vi "Insert Created.vi"(8 "Self":refnum<class "Msg Type Strategy.lvclass">, 9 "Self Alias":string, 10 "Addresses DVR in":refnum<data-value>) -> (0 "error out":errorcluster, 2 "Addresses DVR out":refnum<data-value>)   [LabVIEW 2021, in "jettl.lvlib" / "Addresses.lvlib"]
uses:
  Addresses.lvlib
  Addresses/Addresses.lvclass
  Msg Type Strategy/Msg Type Strategy/Msg Type Strategy.lvclass
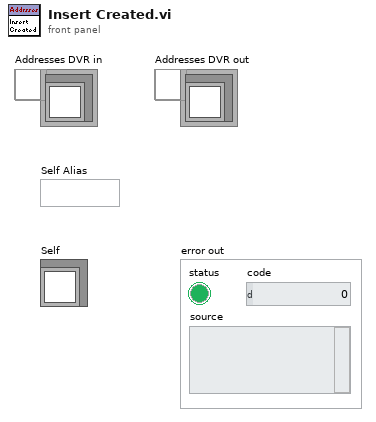
[diagram p1: front panel]
types:
  T1 = typedef "jettl.lvlib/Addresses.lvlib/Created.ctl" = map{string, refnum<class "Msg Type Strategy.lvclass">}
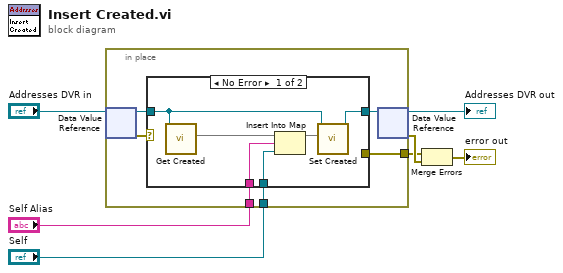
[diagram p0: block diagram]
diagram:
  n1 = in-place {
    in-place-border: [w13] -> w3
    in-place-border: "Self Alias" -> [w10]
    in-place-border: "Self" -> [w8]
    n2 = in-place-dvr #1("Addresses DVR in") -> (w11:refnum<class "Addresses.lvclass">, w12:errorcluster)
    n3 = case shown="No Error" w12 {
      selector: w12 -> [_ w21]
      tunnel: w11 -> [w16 w20]
      tunnel: [_ w21] -> w13
      tunnel: w10 -> [w18 _]
      tunnel: [w15 w20] -> w9
      tunnel: w8 -> [w14 _]
      frame No Error {
        n4 = call "Get Created.vi"("Addresses in"=w16) -> ("Created"=w19:T1)  [unwired: 10 in]
        n5 = Insert Into Map(map in=w19, key=w18, value=w14) -> (map out=w17:T1)  [unwired: 2 out]
        n6 = call "Set Created.vi"("Created"=w17, "Addresses in"=w16) -> ("Addresses out"=w15:refnum<class "Addresses.lvclass">)  [unwired: 9 in]
      }
      frame Error {
      }
    }
    n7 = in-place-dvr #1(w9) -> (→"Addresses DVR out":refnum<data-value>, w4:errorcluster)
  }
  n8 = Merge Errors(w3, w4) -> (→"error out":errorcluster)
